vi "spectrum_test_lx.vi"() -> ()   [LabVIEW 2017]
uses:
  <userlib>/RSA_API/RSA_API.lvlib
panel:
  out "Waveform Graph 2":sgl[](graph)
  out "outTracePoints":i32
  out "ready out":bool=TRUE
  out "span out":dbl
  in  "span":dbl=40000000.0
  in  "enable":bool=TRUE
  out "enable out":bool=TRUE
  out "cf out":dbl
  in  "cf":dbl=1000000000.0
  out "serialNum out":string
  out "numDevicesFound out":i32
  in  "deviceID":i32
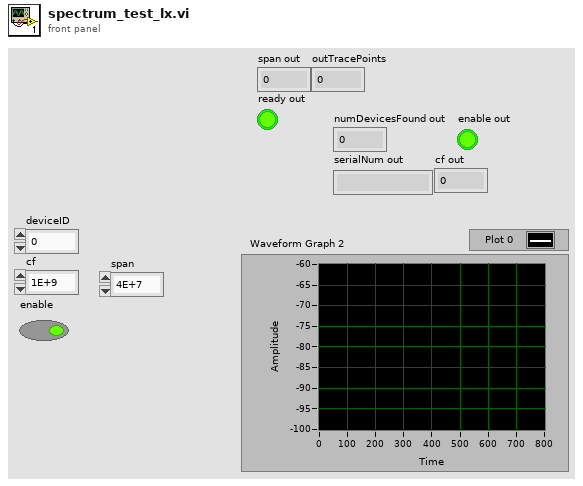
[diagram p1: front panel]
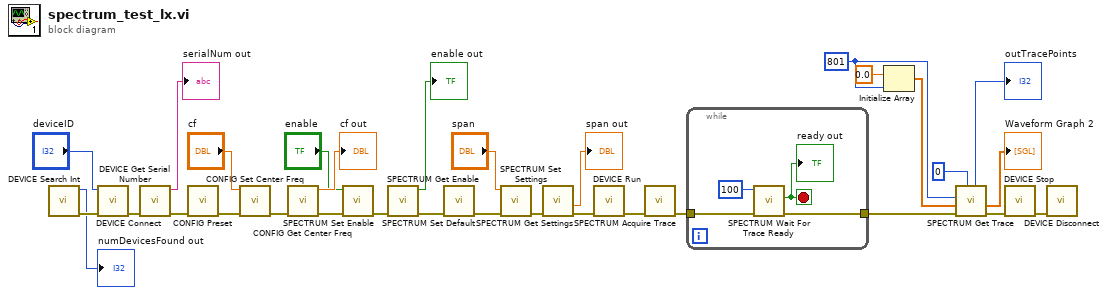
[diagram p0: block diagram]
diagram:
  w3 = 801 ("maxTracePoints")
  n1 = call <userlib>:"DEVICE Search Int.vi"() -> ("error out"=w31:errorcluster, "numDevicesFound out"=→"numDevicesFound out":i32)  [unwired: 8 in, 2 out]
  n2 = call <userlib>:"DEVICE Connect.vi"("error in (no error)"=w31, "deviceID"="deviceID") -> ("error out"=w28:errorcluster)  [unwired: 8 in, 1 out]
  n3 = call <userlib>:"DEVICE Get Serial Number.vi"("error in (no error)"=w28) -> ("error out"=w16:errorcluster, "serialNum out"=→"serialNum out":string)  [unwired: 8 in, 1 out]
  n4 = call <userlib>:"CONFIG Preset.vi"("error in (no error)"=w16) -> ("error out"=w17:errorcluster)  [unwired: 9 in, 1 out]
  n5 = call <userlib>:"CONFIG Set Center Freq.vi"("error in (no error)"=w17, "cf"="cf") -> ("error out"=w25:errorcluster)  [unwired: 8 in, 1 out]
  n6 = call <userlib>:"CONFIG Get Center Freq.vi"("error in (no error)"=w25) -> ("error out"=w21:errorcluster, "cf out"=→"cf out":dbl)  [unwired: 8 in, 1 out]
  n7 = call <userlib>:"SPECTRUM Set Enable.vi"("error in (no error)"=w21, "enable"="enable") -> ("error out"=w20:errorcluster)  [unwired: 8 in, 1 out]
  n8 = call <userlib>:"SPECTRUM Get Enable.vi"("error in (no error)"=w20) -> ("error out"=w18:errorcluster, "enable out"=→"enable out":bool)  [unwired: 8 in, 1 out]
  n9 = call <userlib>:"SPECTRUM Set Default.vi"("error in (no error)"=w18) -> ("error out"=w14:errorcluster)  [unwired: 9 in, 1 out]
  n10 = call <userlib>:"SPECTRUM Set Settings.vi"("error in (no error)"=w14, "span"="span") -> ("error out"=w12:errorcluster)  [unwired: 8 in, 1 out]
  n11 = call <userlib>:"SPECTRUM Get Settings.vi"("error in (no error)"=w12) -> ("error out"=w9:errorcluster, "span"=→"span out":dbl)  [unwired: 8 in, 1 out]
  n12 = call <userlib>:"DEVICE Run.vi"("error in (no error)"=w9) -> ("error out"=w8:errorcluster)  [unwired: 9 in, 1 out]
  n13 = call <userlib>:"SPECTRUM Acquire Trace.vi"("error in (no error)"=w8) -> ("error out"=w7:errorcluster)  [unwired: 9 in, 1 out]
  n14 = while {
    tunnel: w7 -> [w33]
    tunnel: [w32] -> w6
    stop <- w35 stop-if-true
    n15 = call <userlib>:"SPECTRUM Wait For Trace Ready.vi"("error in (no error)"=w33, "timeoutMsec"=100) -> ("error out"=w32:errorcluster, "ready out"=w35:bool)  [unwired: 7 in, 1 out]
    "ready out" <- w35
  }
  n16 = Initialize Array(0.0 ("element"), w3) -> (w4:dbl[])
  n17 = call <userlib>:"SPECTRUM Get Trace.vi"("outTracePoints"=0, "error in (no error)"=w6, "traceData"=w4, "maxTracePoints"=w3) -> ("error out"=w5:errorcluster, "traceData out"=→"Waveform Graph 2":sgl[], "outTracePoints out"=→"outTracePoints":i32)  [unwired: 4 in, 1 out]
  n18 = call <userlib>:"DEVICE Stop.vi"("error in (no error)"=w5) -> ("error out"=w22:errorcluster)  [unwired: 9 in, 1 out]
  n19 = call <userlib>:"DEVICE Disconnect.vi"("error in (no error)"=w22) -> ()  [unwired: 9 in, 2 out]
